vi "test Write and Read Float.vi"(8 "error in (no error)":errorcluster, 11 "TestCase in":refnum<class "Read Value Tests.lvclass">) -> (0 "error out":errorcluster, 3 "TestCase out":refnum<class "Read Value Tests.lvclass">)   [LabVIEW 2017, in "Mem Buff Tests.lvlib" / "Read Value Tests.lvclass"]
uses:
  Read Value Tests.lvclass
  Read Value Tests.lvclass/Read Value Tests.ctl
  Engine/Classes/Buffer/Read 0D SGL.vi
  Engine/Classes/Buffer/Read 0D DBL.vi
  <vilib>/addons/_JKI Toolkits/VI Tester/TestCase.llb/TestCase.lvclass
  Engine/Classes/Buffer/Buffer.lvclass
  C:/Program Files (x86)/National Instruments/LabVIEW 2017/vi.lib/addons/_JKI Toolkits/VI Tester/TestCase.llb/TestCase.lvclass
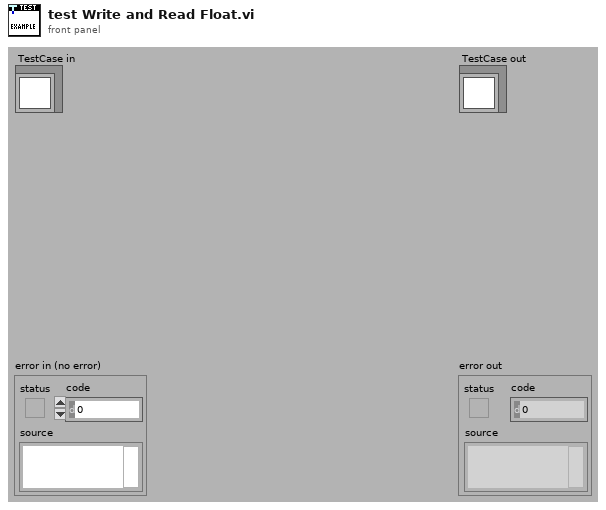
[diagram p1: front panel]
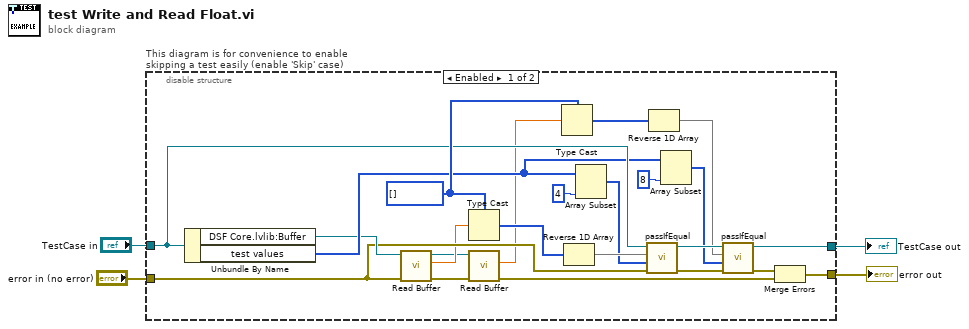
[diagram p0: block diagram]
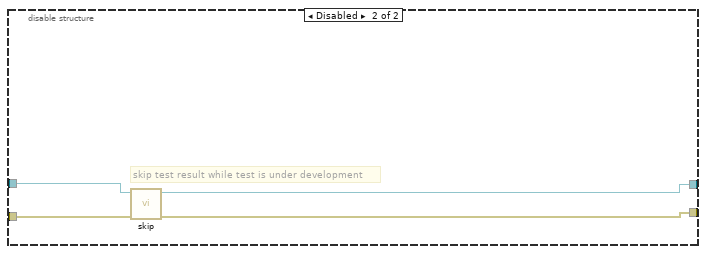
[diagram p2: hidden frame]
diagram:
  n1 = disable-structure "This diagram is for convenience to enable skipping a test easily (enable 'Skip' case)" shown="Enabled" {
    disable-tunnel: "TestCase in" -> [w14 w31]
    disable-tunnel: [w18 w29] -> w1
    disable-tunnel: [w13 w30] -> w2
    disable-tunnel: "error in (no error)" -> [w10 w28]
    frame Enabled {
      w19 = u8[] [] ("buffer in")
      n2 = Unbundle By Name(w14) -> ("DSF Core.lvlib:Buffer"=w11:refnum<class "Buffer.lvclass">, "test values"=w12:u8[])
      n3 = call-poly "Read Buffer.vi"("error in (no error)"=w10, "Buffer in"=w11) -> ("error out"=w7:errorcluster, "value out"=w9:sgl, "Buffer out"=w8:refnum<class "Buffer.lvclass">)  [unwired: 6 in, 1 out]
      n4 = Type Cast(type=w19, x=w9) -> (*(type *) &x=w27:u8[])
      n5 = call-poly "Read Buffer.vi"("error in (no error)"=w7, "Buffer in"=w8) -> ("error out"=w6:errorcluster, "value out"=w5:dbl)  [unwired: 6 in, 2 out]
      n6 = Type Cast(type=w19, x=w5) -> (*(type *) &x=w21:u8[])
      n7 = Reverse 1D Array(array=w27) -> (reversed array=w25:u8[])
      n8 = Array Subset(array=w12, length=4) -> (w16:u8[])  [unwired: 1 in]
      n9 = call-dynamic "passIfEqual.vi"("error in (no error)"=w10, "y"=w16, "x"=w25, "TestCase in"=w14) -> ("error out"=w26:errorcluster, "TestCase out"=w23:refnum<class "Read Value Tests.lvclass">)  [unwired: 6 in]
      n10 = Reverse 1D Array(array=w21) -> (reversed array=w20:u8[])
      n11 = Array Subset(array=w12, length=8) -> (w15:u8[])  [unwired: 1 in]
      n12 = call-dynamic "passIfEqual.vi"("error in (no error)"=w26, "y"=w15, "x"=w20, "TestCase in"=w23) -> ("error out"=w17:errorcluster, "TestCase out"=w18:refnum<class "Read Value Tests.lvclass">)  [unwired: 6 in]
      n13 = Merge Errors(w17, w6) -> (w13:errorcluster)
    }
    frame Disabled {
      # "skip test result while test is under development"
      n14 = call <vilib>:"skip.vi"("error in (no error)"=w28, "TestCase in"=w31) -> ("error out"=w30:errorcluster, "TestCase out"=w29:refnum<class "Read Value Tests.lvclass">)  [unwired: 8 in]
    }
  }
  "error out" <- w2
  "TestCase out" <- w1
